vi "读取CreateEPUBCommand.vi"(8 "error in (no error)":errorcluster caption="错误输入（无错误）", 11 "EPUB输入":refnum<class "EPUB.lvclass">) -> (0 "error out":errorcluster caption="错误输出", 2 "EPUB路径":string, 3 "EPUB输出":refnum<class "EPUB.lvclass">)   [LabVIEW 2016]
uses:
  EPUB.lvclass
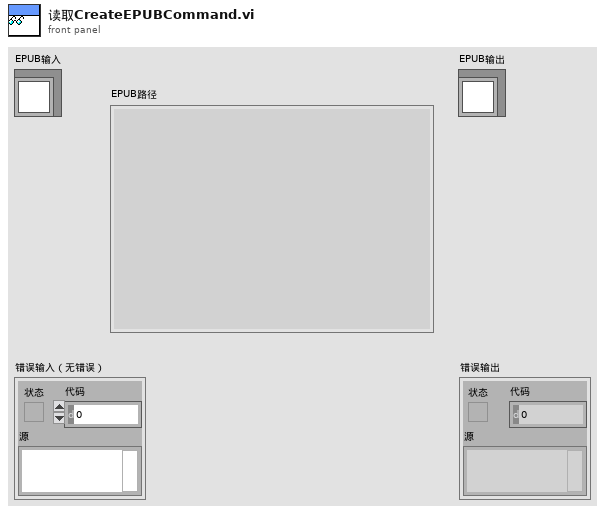
[diagram p1: front panel]
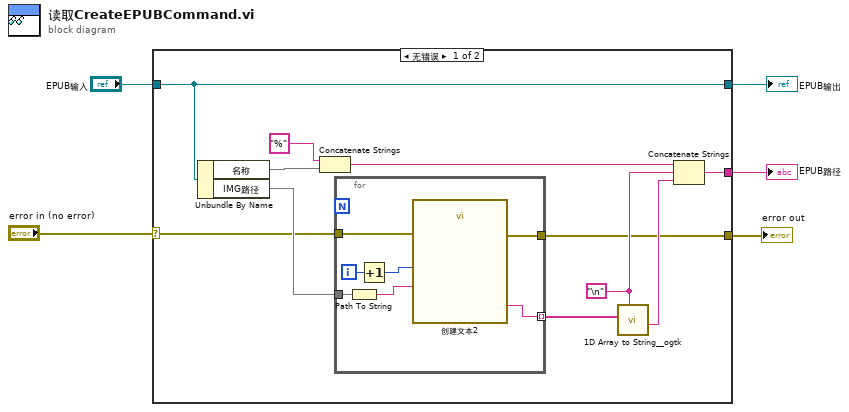
[diagram p0: block diagram]
diagram:
  n1 = case shown="无错误" "error in (no error)" {
    selector: "error in (no error)" -> [w11 w24]
    tunnel: [w6 w24] -> w4
    tunnel: [w16 w25] -> w2
    tunnel: "EPUB输入" -> [w16 w25]
    tunnel: [w10 _] -> w1
    frame No Error {
      w8 = "\n"
      n2 = Unbundle By Name(w16) -> ("名称"=w15, "IMG路径"=w12)
      n3 = Concatenate Strings("%" ("字符串"), w15) -> (w14:string)
      n4 = for {
        tunnel: w12 -> [w22]
        tunnel: w11 -> [w18]
        tunnel: [w19] -> w7 mode=indexing
        tunnel: [w17] -> w6
        i -> [w23]
        n5 = Path To String(path=w22) -> (string=w21:string)
        n6 = Increment(x=w23) -> (x+1=w20:i32)
        n7 = call "创建文本2"("imgidx"=w20, "img"=w21, "error in (no error)"=w18) -> ("Result"=w19:string, "error out"=w17:errorcluster)  [unwired: 11 in]
      }
      n8 = call <userlib>:"1D Array to String__ogtk.vi"("delimiter (Tab)"=w8, "Array of Strings"=w7) -> ("delimited string"=w9:string)  [unwired: 9 in]
      n9 = Concatenate Strings(w14, w8, w9) -> (w10:string)
    }
    frame Error {
    }
  }
  "error out" <- w4
  "EPUB输出" <- w2
  "EPUB路径" <- w1
